vi "color checking.vi"(0 "Color list":string[][](array[string]), 3 "Image in":T2(plugin-control), 7 "error in":errorcluster) -> (20 "Image Out":T2(plugin-control), 23 "Color Result":T1(array[cluster]), 27 "error out":errorcluster)   [LabVIEW 2020]
uses:
  <vilib>/vision/NI_Vision_Development_Module.lvlib
panel:
  out "Array 2":i32[](array[numeric])
  out "Array":bool[](array[boolean])
  out "Match Score (Color Matching 1)":i32[](array[numeric])
  out "Match Flag (Color Matching 1)":bool[](array[boolean])
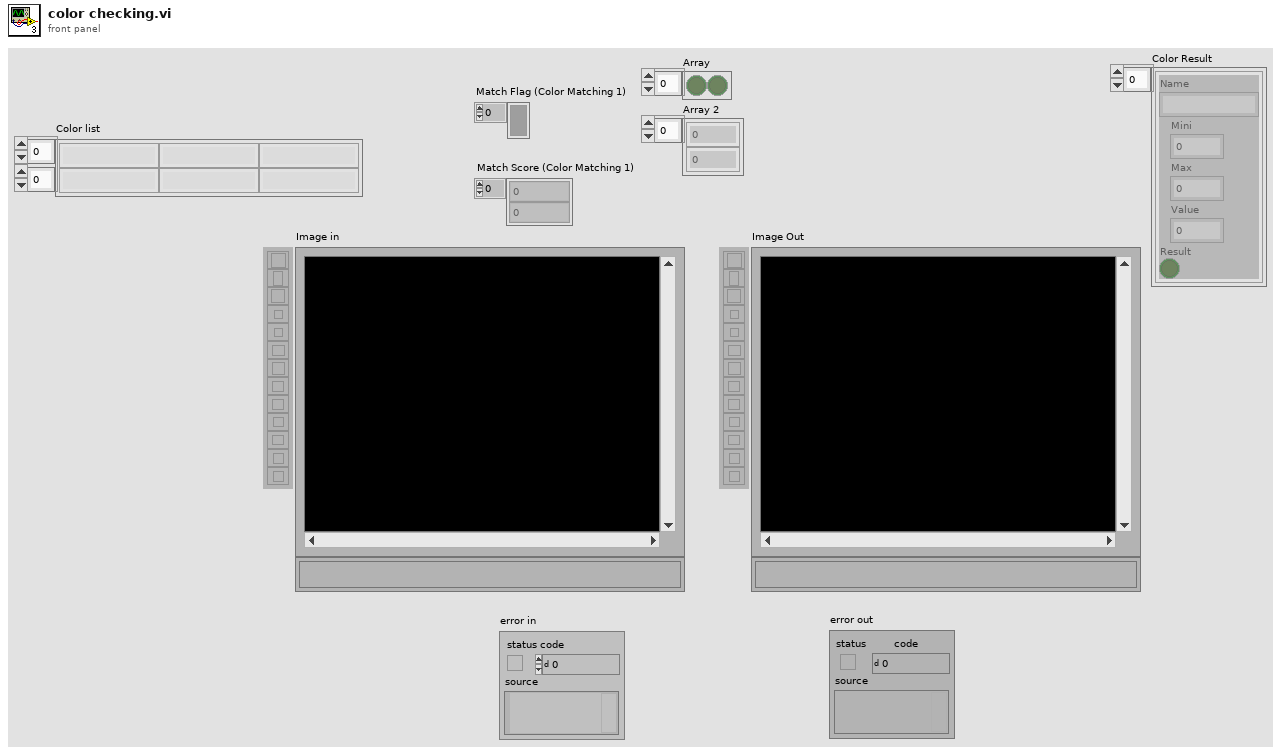
[diagram p1: front panel]
types:
  T1 = cluster{"Name":string, "Mini":dbl, "Max":dbl, "Value ":dbl, "Result":bool}[]
  T2 = typedef "IMAQ Image.ctl" = refnum<image>
  T3 = cluster{"Name":string, "Mini":dbl, "Max":dbl, "Value ":dbl, "Result":bool}
  T4 = cluster{"Global Rectangle":i32[], "Contours":cluster{"Contour Type":u32, "ROI Type":u32, "Points":i32[]}[]}
  T5 = typedef "ROI Descriptor" = cluster{"Global Rectangle":i32[], "Contours":cluster{"ID":enum32{"External", "Internal"}, "Type":u32, "Coordinates":i32[]}[]}
  T6 = typedef "Image Type" = u32
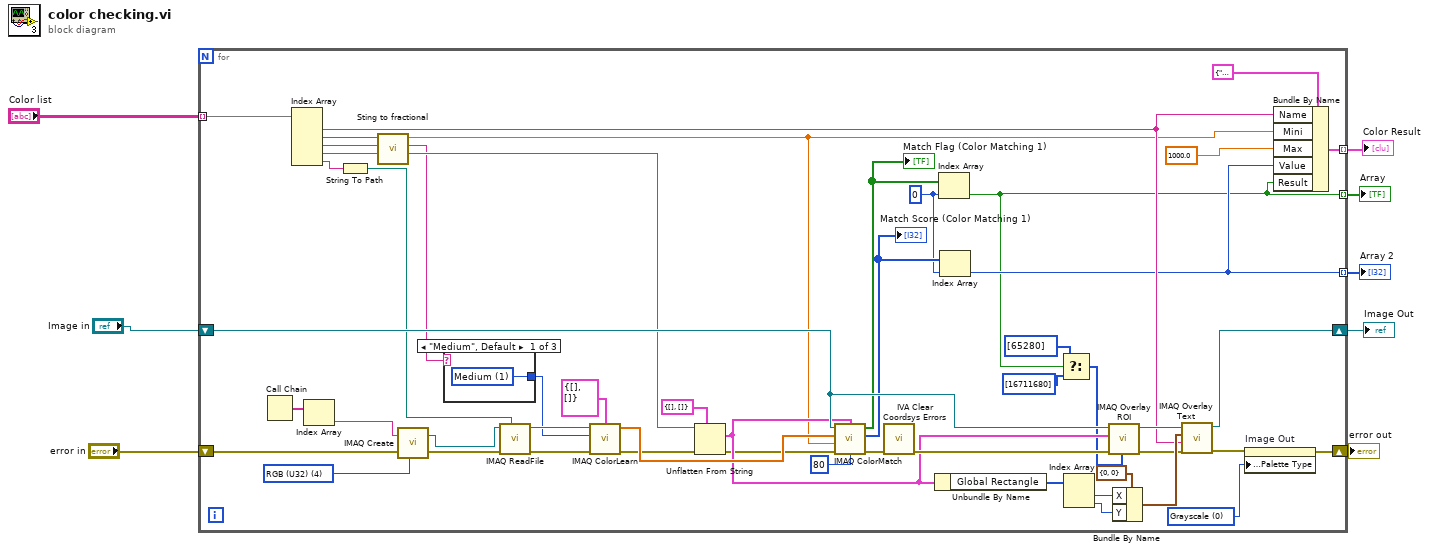
[diagram p0: block diagram]
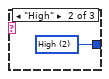
[diagram p2: hidden frame]
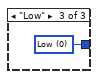
[diagram p3: hidden frame]
diagram:
  n1 = for {
    shift-right: [w50] -> w7
    shift-left: "error in" -> [w55]
    tunnel: "Color list" -> [w39] mode=indexing
    shift-right: [w37] -> w4
    shift-left: "Image in" -> [w40]
    tunnel: [w12] -> w3 mode=indexing
    tunnel: [w13] -> w2 mode=indexing
    tunnel: [w14] -> w1 mode=indexing
    w20 = 0 ("index")
    w49 = u32 0 items=["Grayscale", "Binary", "Gradient", "Rainbow", "Temperature", "User Defined", "Binary 16 Bit", "Gradient 16 Bit", "Rainbow 16 Bit", "Temperature 16 Bit", "User Defined 16 Bit"] ("Palette Type")
    w52 = T6 4 items=["Grayscale (U8)", "Grayscale (I16)", "Grayscale (SGL)", "Complex (CSG)", "RGB (U32)", "HSL (U32)", "RGB (U64)", "Grayscale (U16)"] ("Image Type")
    n2 = Call Chain() -> (call chain=w54:string[])
    n3 = Index Array(array=w39) -> (element #1=w17:string, element #2=w28:string, element #3=w19:string, element #4=w25:string, element #5=w24:string)  [unwired: 5 in]
    n4 = Index Array(array=w54) -> (element=w53:string)  [unwired: 1 in]
    n5 = String To Path(string=w24) -> (path=w23:path)
    n6 = call "Sting to fractional.vi"("String"=w28) -> ("Numeric"=w16:dbl)  [unwired: 10 in]
    n7 = call "IMAQ Create"("Image Name"=w53, "Image Type"=w52, "error in (no error)"=w55) -> ("New Image"=w57:T2, "error out"=w56:errorcluster)  [unwired: 1 in, 1 out]
    n8 = case shown="\"Medium\", Default" w19 {
      tunnel: [w58 w59 w60] -> w42
      frame "Medium", Default {
        w58 = u32 1 items=["Low", "Medium", "High"] ("Color Sensitivity")
      }
      frame "High" {
        w59 = u32 2 items=["Low", "Medium", "High"] ("Color Sensitivity")
      }
      frame "Low" {
        w60 = u32 0 items=["Low", "Medium", "High"] ("Color Sensitivity")
      }
    }
    n9 = call "IMAQ ReadFile"("File Path"=w23, "error in (no error)"=w56, "Image"=w57) -> ("error out"=w44:errorcluster, "Image Out"=w46:T2)  [unwired: 2 in, 5 out]
    n10 = call "IMAQ ColorLearn"("ROI Descriptor"=T5 {"Global Rectangle"=[], "Contours"=[]}, "Image"=w46, "Color Sensitivity"=w42, "error in (no error)"=w44) -> ("Color Spectrum"=w48:dbl[], "error out"=w27:errorcluster)  [unwired: 4 in]
    n11 = Unflatten From String(type=T4 {"Global Rectangle"=[], "Contours"=[]} ("ROI"), binary string=w25, error in (no error)=w27) -> (value=w33:T4, error out=w26:errorcluster)  [unwired: 2 in, 1 out]
    n12 = call "IMAQ ColorMatch"("ROI Descriptor"=w33, "Image"=w40, "Color Spectrum"=w48, "Match Saturation Threshold"=80, "Minimum Match Score"=w16, "error in (no error)"=w26) -> ("Match Flag"=w22:bool[], "Match Score"=w21:i32[], "error out"=w51:errorcluster)  [unwired: 1 out]
    "Match Flag (Color Matching 1)" <- w22
    "Match Score (Color Matching 1)" <- w21
    n13 = call <vilib>:"IVA Clear Coordsys Errors.vi"("error in (no error)"=w51) -> ("error out"=w47:errorcluster)  [unwired: 10 in]
    n14 = Unbundle By Name(w33) -> ("Global Rectangle"=w32:i32[])
    n15 = Index Array(array=w22, index=w20) -> (element=w12:bool)
    n16 = Index Array(array=w21, index=w20) -> (element=w13:i32)
    n17 = Select(t=u32[] [65280] ("Colors (Green)"), s=w12, f=u32[] [16711680] ("Colors (Green)")) -> (s? t:f=w9:u32[])
    n18 = Index Array(array=w32) -> (element #1=w35:i32, element #2=w34:i32)  [unwired: 2 in]
    n19 = call "IMAQ Overlay ROI"("Colors (Green)"=w9, "error in (no error)"=w47, "ROI Descriptor"=w33, "Image"=w40) -> ("error out"=w30:errorcluster, "Image Out"=w38:T2)  [unwired: 6 in]
    n20 = Bundle By Name(cluster=cluster{"X":i32, "Y":i32} {"X"=0, "Y"=0}, "X"=w35, "Y"=w34) -> (w31:cluster{"X":i32, "Y":i32})
    n21 = call "IMAQ Overlay Text"("error in (no error)"=w30, "String"=w17, "Origin"=w31, "Image"=w38) -> ("error out"=w29:errorcluster, "Image Out"=w37:T2)  [unwired: 6 in]
    n22 = property on="Image Out" class="ImageControl"(error in=w29, "Palette:Palette Type"=w49) -> (error out=w50:errorcluster)  [unwired: 1 in, 1 out]
    n23 = Bundle By Name(cluster=T3 {"Name"="", "Mini"=0.0, "Max"=0.0, "Value "=0.0, "Result"=FALSE}, "Name"=w17, "Mini"=w16, "Max"=1000.0, "Value"=w13, "Result"=w12) -> (w14:T3)
  }
  "error out" <- w7
  "Image Out" <- w4
  "Array" <- w3
  "Array 2" <- w2
  "Color Result" <- w1
